vi "Initialise.vi"(8 "error in (no error)":errorcluster, 10 "Config Name":string, 11 "Config Directory":path) -> (0 "error out":errorcluster)   [LabVIEW 2015, in "System Config.lvclass"]
uses:
  System Config.lvclass
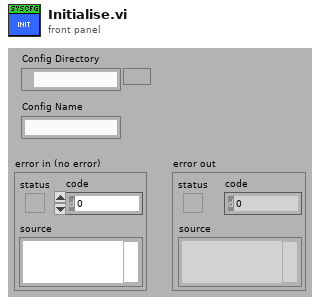
[diagram p1: front panel]
types:
  T1 = typedef "System Config.lvclass/ClassAttributesRef.ctl" = refnum<data-value>
  T2 = typedef "System Config.lvclass/ClassAttributes.ctl" = cluster{"Config":cluster{"Logging":cluster{"Log Files Directory":path, "Max Lines Per Log File":i32}, "Settings":T3}, "Core":cluster{"Config Directory":path, "Name":string, "Config Changed":refnum<user-event>}}
  T3 = typedef "System Config.lvclass/Settings.ctl" = cluster{"Dummy":dbl}
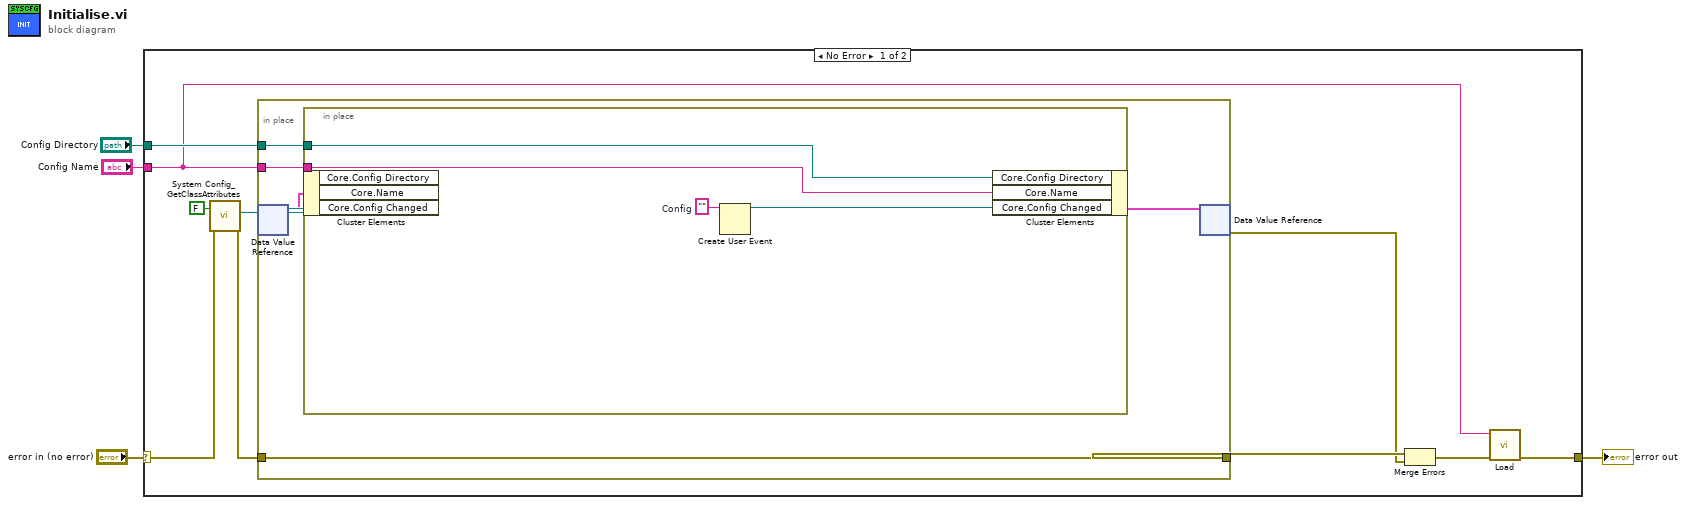
[diagram p0: block diagram]
diagram:
  n1 = case shown="No Error" "error in (no error)" {
    selector: "error in (no error)" -> [w14 w24]
    tunnel: [w6 w24] -> w3
    tunnel: "Config Name" -> [w5 _]
    tunnel: "Config Directory" -> [w8 _]
    frame No Error {
      n2 = call "System Config_GetClassAttributes.vi"("error in (no error)"=w14, "return data? (T)"=FALSE ("return data")) -> ("error out"=w13:errorcluster, "class attributes ref"=w12:T1)  [unwired: 6 in, 2 out]
      n3 = in-place {
        in-place-border: w13 -> [w17]
        in-place-border: [w17] -> w10
        in-place-border: w5 -> [w16]
        in-place-border: w8 -> [w15]
        n4 = in-place-dvr #1(w12) -> (w18:T2)  [unwired: 1 out]
        n5 = in-place {
          in-place-border: w16 -> [w21]
          in-place-border: w15 -> [w20]
          w23 = ""  # Config
          n6 = in-place-cluster #2(w18) -> ()  [unwired: 3 out]
          n7 = Create User Event(user event datatype=w23) -> (user event=w22:refnum<user-event>)  [unwired: 1 in, 1 out]
          n8 = in-place-cluster #2("Core.Config Directory"=w20, "Core.Name"=w21, "Core.Config Changed"=w22) -> (w19:T2)
        }
        n9 = in-place-dvr #1(w19) -> (w9:errorcluster)  [unwired: 1 out]
      }
      n10 = Merge Errors(w10, w9) -> (w7:errorcluster)
      n11 = call "Load.vi"("error in (no error)"=w7, "Config Name"=w5) -> ("error out"=w6:errorcluster)  [unwired: 9 in]
    }
    frame Error {
    }
  }
  "error out" <- w3
